vi "createScanArrays.vi"(4 "error in":errorcluster, 7 "resolution":i32=4 min=4 max=2048 step=2) -> (0 "error out":errorcluster, 2 "y-array":dbl[](array[numeric]), 3 "x-array":dbl[](array[numeric]))   [LabVIEW 2015]
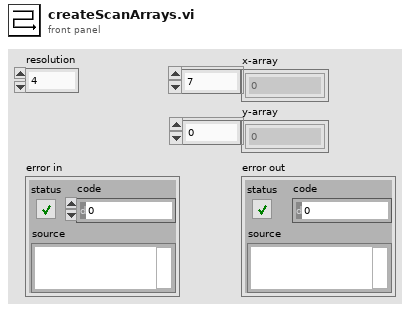
[diagram p1: front panel]
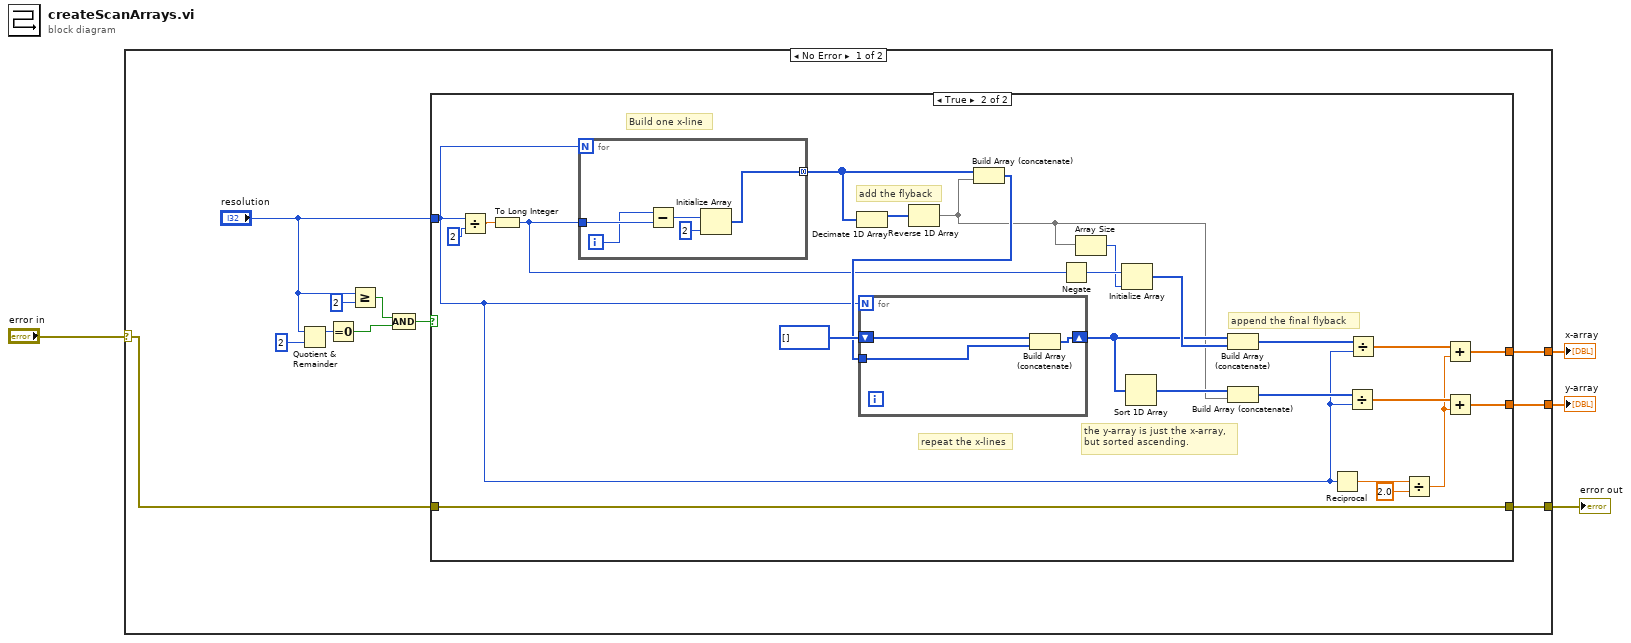
[diagram p0: block diagram]
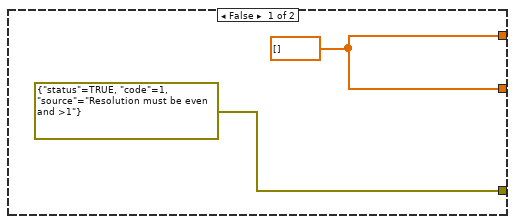
[diagram p2: hidden frame]
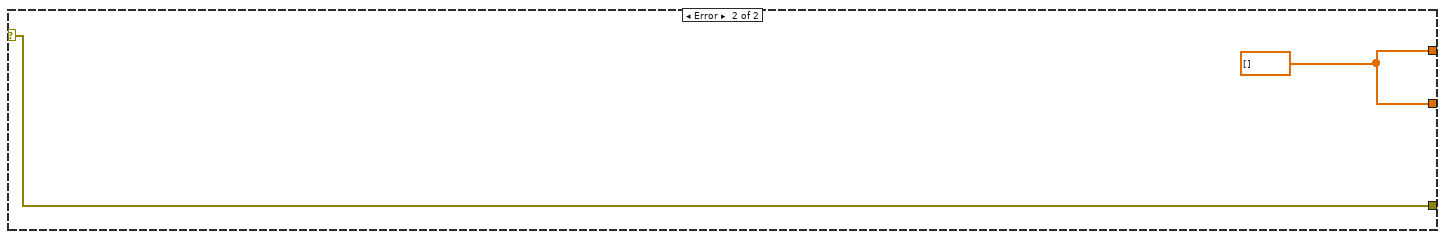
[diagram p3: hidden frame]
diagram:
  n1 = case shown="No Error" "error in" {
    selector: "error in" -> [w7 w51]
    tunnel: [w8 w51] -> w4
    tunnel: [w6 w50] -> w2
    tunnel: [w5 w50] -> w1
    frame No Error {
      n2 = Quotient & Remainder(x="resolution", y=2) -> (x-y*floor(x/y)=w14:i32)  [unwired: 1 out]
      n3 = Equal To 0?(x=w14) -> (x = 0?=w13:bool)
      n4 = Greater Or Equal?(x="resolution", y=2) -> (x >= y?=w9:bool)
      n5 = Compound Arithmetic op=AND(w9, w13) -> (w12:bool)
      n6 = case shown="True" w12 {
        tunnel: "resolution" -> [_ w21]
        tunnel: [errorcluster {"status"=TRUE, "code"=1, "source"="Resolution must be even and >1"} ("error constant") w34] -> w8
        tunnel: w7 -> [_ w34]
        tunnel: [w16 w23] -> w6
        tunnel: [w16 w22] -> w5
        frame False {
          w16 = dbl[] []
        }
        frame True {
          # "add the flyback"
          # "append the final flyback"
          # "the y-array is just the x-array,\nbut sorted ascending."
          # "repeat the x-lines"
          # "Build one x-line"
          n7 = Divide(x=w21, y=2) -> (x/y=w28:dbl)
          n8 = To Long Integer(number=w28) -> (32bit integer=w27:i32)
          n9 = for {
            N: w21 -> [_]
            tunnel: w27 -> [w49]
            tunnel: [w45] -> w26 mode=concatenating
            i -> [w48]
            n10 = Subtract(x=w48, y=w49) -> (x-y=w46:i32)
            n11 = Initialize Array(w46, 2 ("dimension size")) -> (w45:i32[])
          }
          n12 = Decimate 1D Array(w26) -> (w25:i32[])  [unwired: 1 out]
          n13 = Reverse 1D Array(array=w25) -> (reversed array=w24:i32[])
          n14 = Build Array (concatenate)(w26, w24) -> (w29:i32[])
          n15 = for {
            N: w21 -> [_]
            tunnel: w29 -> [w43]
            shift-right: [w42] -> w35
            shift-left: i32[] [] -> [w44]
            n16 = Build Array (concatenate)(w44, w43) -> (w42:i32[])
          }
          n17 = Negate(x=w27) -> (-x=w38:i32)
          n18 = Array Size(array=w24) -> (size(s)=w37:i32)
          n19 = Initialize Array(w38, w37) -> (w36:i32[])
          n20 = Sort 1D Array(array=w35) -> (sorted array=w39:i32[])
          n21 = Build Array (concatenate)(w35, w36) -> (w33:i32[])
          n22 = Build Array (concatenate)(w39, w24) -> (w31:i32[])
          n23 = Reciprocal(x=w21) -> (1/x=w20:dbl)
          n24 = Divide(x=w31, y=w21) -> (x/y=w30:dbl[])
          n25 = Divide(x=w33, y=w21) -> (x/y=w32:dbl[])
          n26 = Divide(x=w20, y=2.0) -> (x/y=w19:dbl)
          n27 = Add(x=w32, y=w19) -> (x+y=w23:dbl[])
          n28 = Add(x=w30, y=w19) -> (x+y=w22:dbl[])
        }
      }
    }
    frame Error {
      w50 = dbl[] []
    }
  }
  "error out" <- w4
  "x-array" <- w2
  "y-array" <- w1
